vi "reward_behavior_phase1.vi"() -> ()   [LabVIEW 2019]
doc: "The myRIO Project template acquires acceleration data from the onboard accelerometer and displays the changes of acceleration values in a waveform chart."
uses:
  <vilib>/Analysis/Matrix/Datatypes/RealMatrix.ctl
  <vilib>/myRIO/Common/Instrument Driver Framework/myRIO v1.0/Encoder/typedefs/Encoder Signal Mode.ctl
  <vilib>/myRIO/Instrument Drivers/Onboard IO/Encoder/typedefs/Encoder Reference.ctl
  <vilib>/myRIO/Common/Instrument Driver Framework/Utilities/typedefs/myRIO Generic Hardware Reference.ctl
  <vilib>/myRIO/Common/Instrument Driver Framework/Utilities/typedefs/Hardware Version Enum.ctl
  <vilib>/myRIO/Common/Instrument Driver Framework/Utilities/typedefs/myRIO v1.0 Reference.ctl
  <vilib>/myRIO/Common/Instrument Driver Framework/Utilities/typedefs/Generic FPGA Reference.ctl
  <vilib>/myRIO/Common/Instrument Driver Framework/myRIO v1.0/Encoder/typedefs/Encoder Channels Enum.ctl
  <vilib>/myRIO/Common/Instrument Driver Framework/myRIO v1.0/Encoder/typedefs/Encoder Configuration v1.0.ctl
  <vilib>/userdefined/High Color/nirio_resource_hc.ctl
  <vilib>/myRIO/Instrument Drivers/Onboard IO/DIO/typedefs/DIO Reference.ctl
  <vilib>/myRIO/Common/Instrument Driver Framework/myRIO v1.0/DIO/typedefs/DIO Channels List.ctl
  <vilib>/myRIO/Common/Instrument Driver Framework/myRIO v1.0/DIO/typedefs/DIO Channels Enum.ctl
  <vilib>/myRIO/Common/Instrument Driver Framework/Utilities/vis/Is FPGA Ref Available.vi
  <vilib>/myRIO/Common/Instrument Driver Framework/myRIO v1.0/Encoder/vis/myRIO v1.1 Open Encoder.vi
  <vilib>/myRIO/Instrument Drivers/Onboard IO/Encoder/vis/Read.vi
  <vilib>/myRIO/Common/Instrument Driver Framework/myRIO v1.0/DIO/vis/myRIO v1.1 Open DIO.vi
  <vilib>/myRIO/Instrument Drivers/Onboard IO/DIO/vis/Write.vi
  <vilib>/myRIO/Instrument Drivers/Onboard IO/DIO/vis/Read.vi
  <vilib>/myRIO/Common/Instrument Driver Framework/Utilities/vis/Validate Channels.vi
  <vilib>/myRIO/Common/Instrument Driver Framework/myRIO v1.0/Encoder/vis/myRIO v1.0 Reserve Encoder.vi
  <vilib>/myRIO/Common/Instrument Driver Framework/myRIO v1.0/DIO/vis/myRIO v1.0 Reserve DIO.vi
  <vilib>/myRIO/Common/Instrument Driver Framework/myRIO v1.0/Encoder/vis/myRIO v1.0 Build MUX Configuration Encoder.vi
  <vilib>/myRIO/Common/Instrument Driver Framework/myRIO v1.0/Resource Manager/vis/myRIO v1.0 Reserve Channel List.vi
  <vilib>/myRIO/Common/Instrument Driver Framework/myRIO v1.0/DIO/vis/myRIO v1.0 Build MUX Configuration DIO.vi
  <vilib>/myRIO/Common/Instrument Driver Framework/myRIO v1.0/Resource Manager/vis/myRIO v1.0 Create Configuration List.vi
  <vilib>/myRIO/Common/Instrument Driver Framework/myRIO v1.0/Resource Manager/vis/myRIO v1.0 Reserve Channel.vi
  <vilib>/myRIO/Common/Instrument Driver Framework/myRIO v1.0/Resource Manager/vis/myRIO v1.0 Unreserve Channel.vi
  <vilib>/myRIO/Common/Instrument Driver Framework/myRIO v1.0/Resource Manager/vis/myRIO v1.0 Build Mutex Name.vi
  <vilib>/Utility/VariantDataType/GetNumericInfo.vi
  <vilib>/Utility/error.llb/Error Cluster From Error Code.vi
  <vilib>/myRIO/Common/Instrument Driver Framework/myRIO v1.0/myRIO v1.1 Open.vi
  <vilib>/myRIO/Common/Instrument Driver Framework/Utilities/vis/IO Manager.vi
  <vilib>/myRIO/Common/Instrument Driver Framework/Utilities/vis/Configuration Manager.vi
  <vilib>/myRIO/Common/Instrument Driver Framework/myRIO v1.0/Resource Manager/vis/myRIO v1.0 Configure IO.vi
  <vilib>/myRIO/Common/Instrument Driver Framework/myRIO v1.0/myRIO v1.0 Close.vi
  <vilib>/myRIO/Common/Instrument Driver Framework/myRIO v1.0/Encoder/vis/myRIO v1.0 Configure Encoder.vi
  <vilib>/myRIO/Common/Instrument Driver Framework/myRIO v1.0/Encoder/vis/myRIO v1.0 Read Encoder.vi
  <vilib>/myRIO/Common/Instrument Driver Framework/myRIO v1.0/DIO/vis/myRIO v1.0 Read DIO.vi
  <vilib>/myRIO/Common/Instrument Driver Framework/myRIO v1.0/DIO/vis/myRIO v1.0 Write DIO.vi
  <vilib>/myRIO/Express VI/Onboard IO/Encoder/Encoder Express VI.xnode
  <vilib>/myRIO/Instrument Drivers/Onboard IO/Encoder/vis/myRIO Encoder Open.xnode
  <vilib>/myRIO/Express VI/Onboard IO/DI/DI Express VI.xnode
  <vilib>/myRIO/Instrument Drivers/Onboard IO/DIO/vis/myRIO DIO Open.xnode
  <vilib>/myRIO/Express VI/Onboard IO/DO/DO Express VI.xnode
  <vilib>/myRIO/Instrument Drivers/Onboard IO/Encoder/Encoder.lvlib
  <vilib>/myRIO/Instrument Drivers/Onboard IO/DIO/DIO.lvlib
  <vilib>/Analysis/Matrix/NI_Matrix.lvlib
panel:
  out "Rewarded trials":dbl[](array[numeric])
  out "Rewards":u16
  out "Active Trial":bool
  out "Array temp2":T1
  out "Stimuli Loaded":bool
  out "Stim_ID":dbl[](array[numeric])
  out "Reward_mat":dbl[](array[numeric])
  out "Reward":bool=TRUE
  out "Frame clock":i32
  out "Licks":u32
  out "Lick":bool
  out "Time":dbl
  out "Stop":bool
  in  "Frames to collect":u32
  out "Overflow?":bool
  out "Counter Value":i32
  out "Velocity":dbl
  out "Velocity Plot":dbl[](graph)
  out "Velocity array":dbl[](array[numeric])
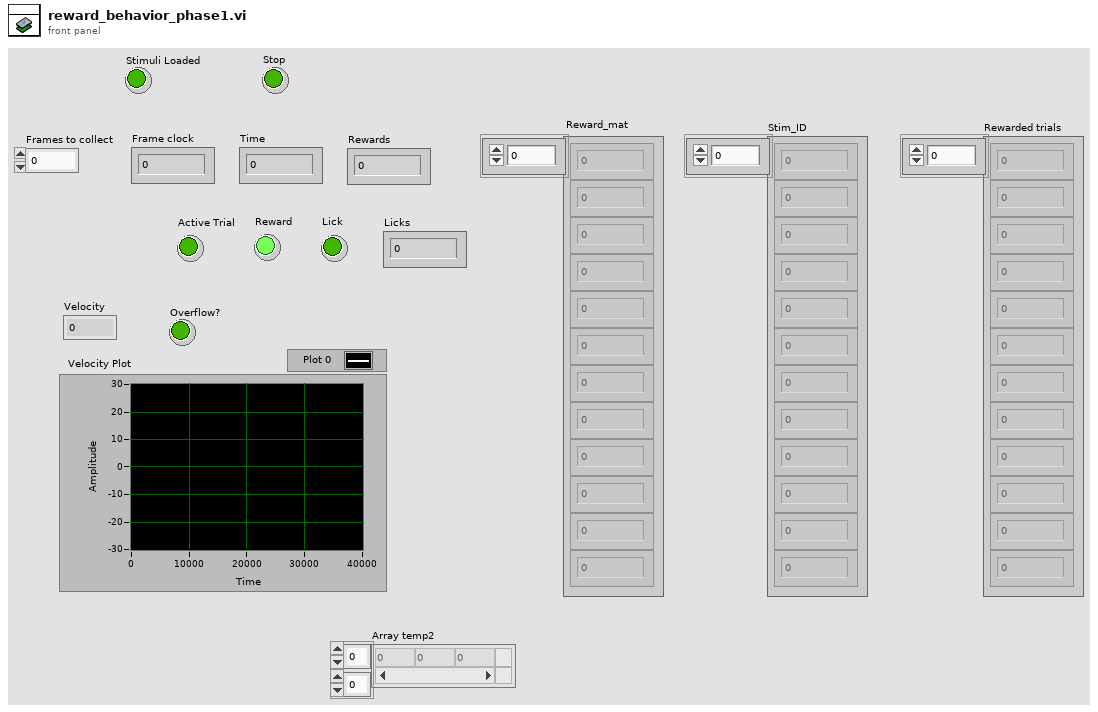
[diagram p1: front panel]
types:
  T1 = typedef "NI_Matrix.lvlib/RealMatrix.ctl" = dbl[][]
  T2 = typedef "Encoder.lvlib/Encoder Reference.ctl" = cluster{"myRIO Reference":T3, "Encoder Channels Enum":T7}
  T3 = typedef "myRIO Generic Hardware Reference.ctl" = cluster{"myRIO Model":T4, "myRIO Hardware Reference":T5}
  T4 = typedef "Hardware Version Enum.ctl" = enum16{"Unknown", "myRIO-1900", "myRIO-1950", "roboRIO", "NI ELVIS RIO CM", "ELVIS III"}
  T5 = typedef "myRIO v1.0 Reference.ctl" = cluster{"Generic FPGA Reference":T6, "Allow multiple opens":bool}
  T6 = typedef "Generic FPGA Reference.ctl" = refnum<k20>
  T7 = typedef "Encoder Channels Enum.ctl" = enum16{"Not Connected", "C/ENC0", "C/ENC1", "A/ENC", "A/ENC0", "A/ENC1", "A/ENC2", "A/ENC3", "A/ENC4", "A/ENC5", "A/ENC6", "A/ENC7", "A/ENC8", "A/ENC9", "B/ENC", "B/ENC0", "B/ENC1", "B/ENC2", "B/ENC3", "B/ENC4", "B/ENC5", "B/ENC6", "B/ENC7", "B/ENC8", "B/ENC9", "DIO/ENC0", "DIO/ENC1", "DIO/ENC2", "DIO/ENC3", "DIO/ENC4"}
  T8 = typedef "Encoder Signal Mode.ctl" = enum16{"Quadrature phase signal", "Step and direction signal"}
  T9 = typedef "nirio_resource_hc.ctl" = tag
  T10 = typedef "DIO.lvlib/DIO Reference.ctl" = cluster{"myRIO Reference":T3, "DIO Channels List":T11}
  T11 = typedef "DIO Channels List.ctl" = T12[]
  T12 = typedef "DIO Channels Enum.ctl" = enum16{"Not Connected", "C/DIO0", "C/DIO1", "C/DIO2", "C/DIO3", "C/DIO4", "C/DIO5", "C/DIO6", "C/DIO7", "A/DIO0", "A/DIO1", "A/DIO2", "A/DIO3", "A/DIO4", "A/DIO5", "A/DIO6", "A/DIO7", "A/DIO8", "A/DIO9", "A/DIO10", "A/DIO11", "A/DIO12", "A/DIO13", "A/DIO14", "A/DIO15", "A/DIO16", "A/DIO17", "A/DIO18", "A/DIO19", "B/DIO0", "B/DIO1", "B/DIO2", "B/DIO3", "B/DIO4", "B/DIO5", "B/DIO6", "B/DIO7", "B/DIO8", "B/DIO9", "B/DIO10", "B/DIO11", "B/DIO12", "B/DIO13", "B/DIO14", "B/DIO15", "B/DIO16", "B/DIO17", "B/DIO18", "B/DIO19", "LED0", "LED1", "LED2", "LED3", "Button0", "DIO/DIO0", "DIO/DIO1", "DIO/DIO2", "DIO/DIO3", "DIO/DIO4", "DIO/DIO5", "DIO/DIO6", "DIO/DIO7", "DIO/DIO8", "DIO/DIO9", "SPI/CS0", "SPI/CS1", "SPI/CS2", "SPI/CS3", "LED RADIO (Green)", "LED RADIO (Red)", "LED COMM (Green)", "LED COMM (Red)", "LED MODE (Green)", "LED MODE (Red)"}
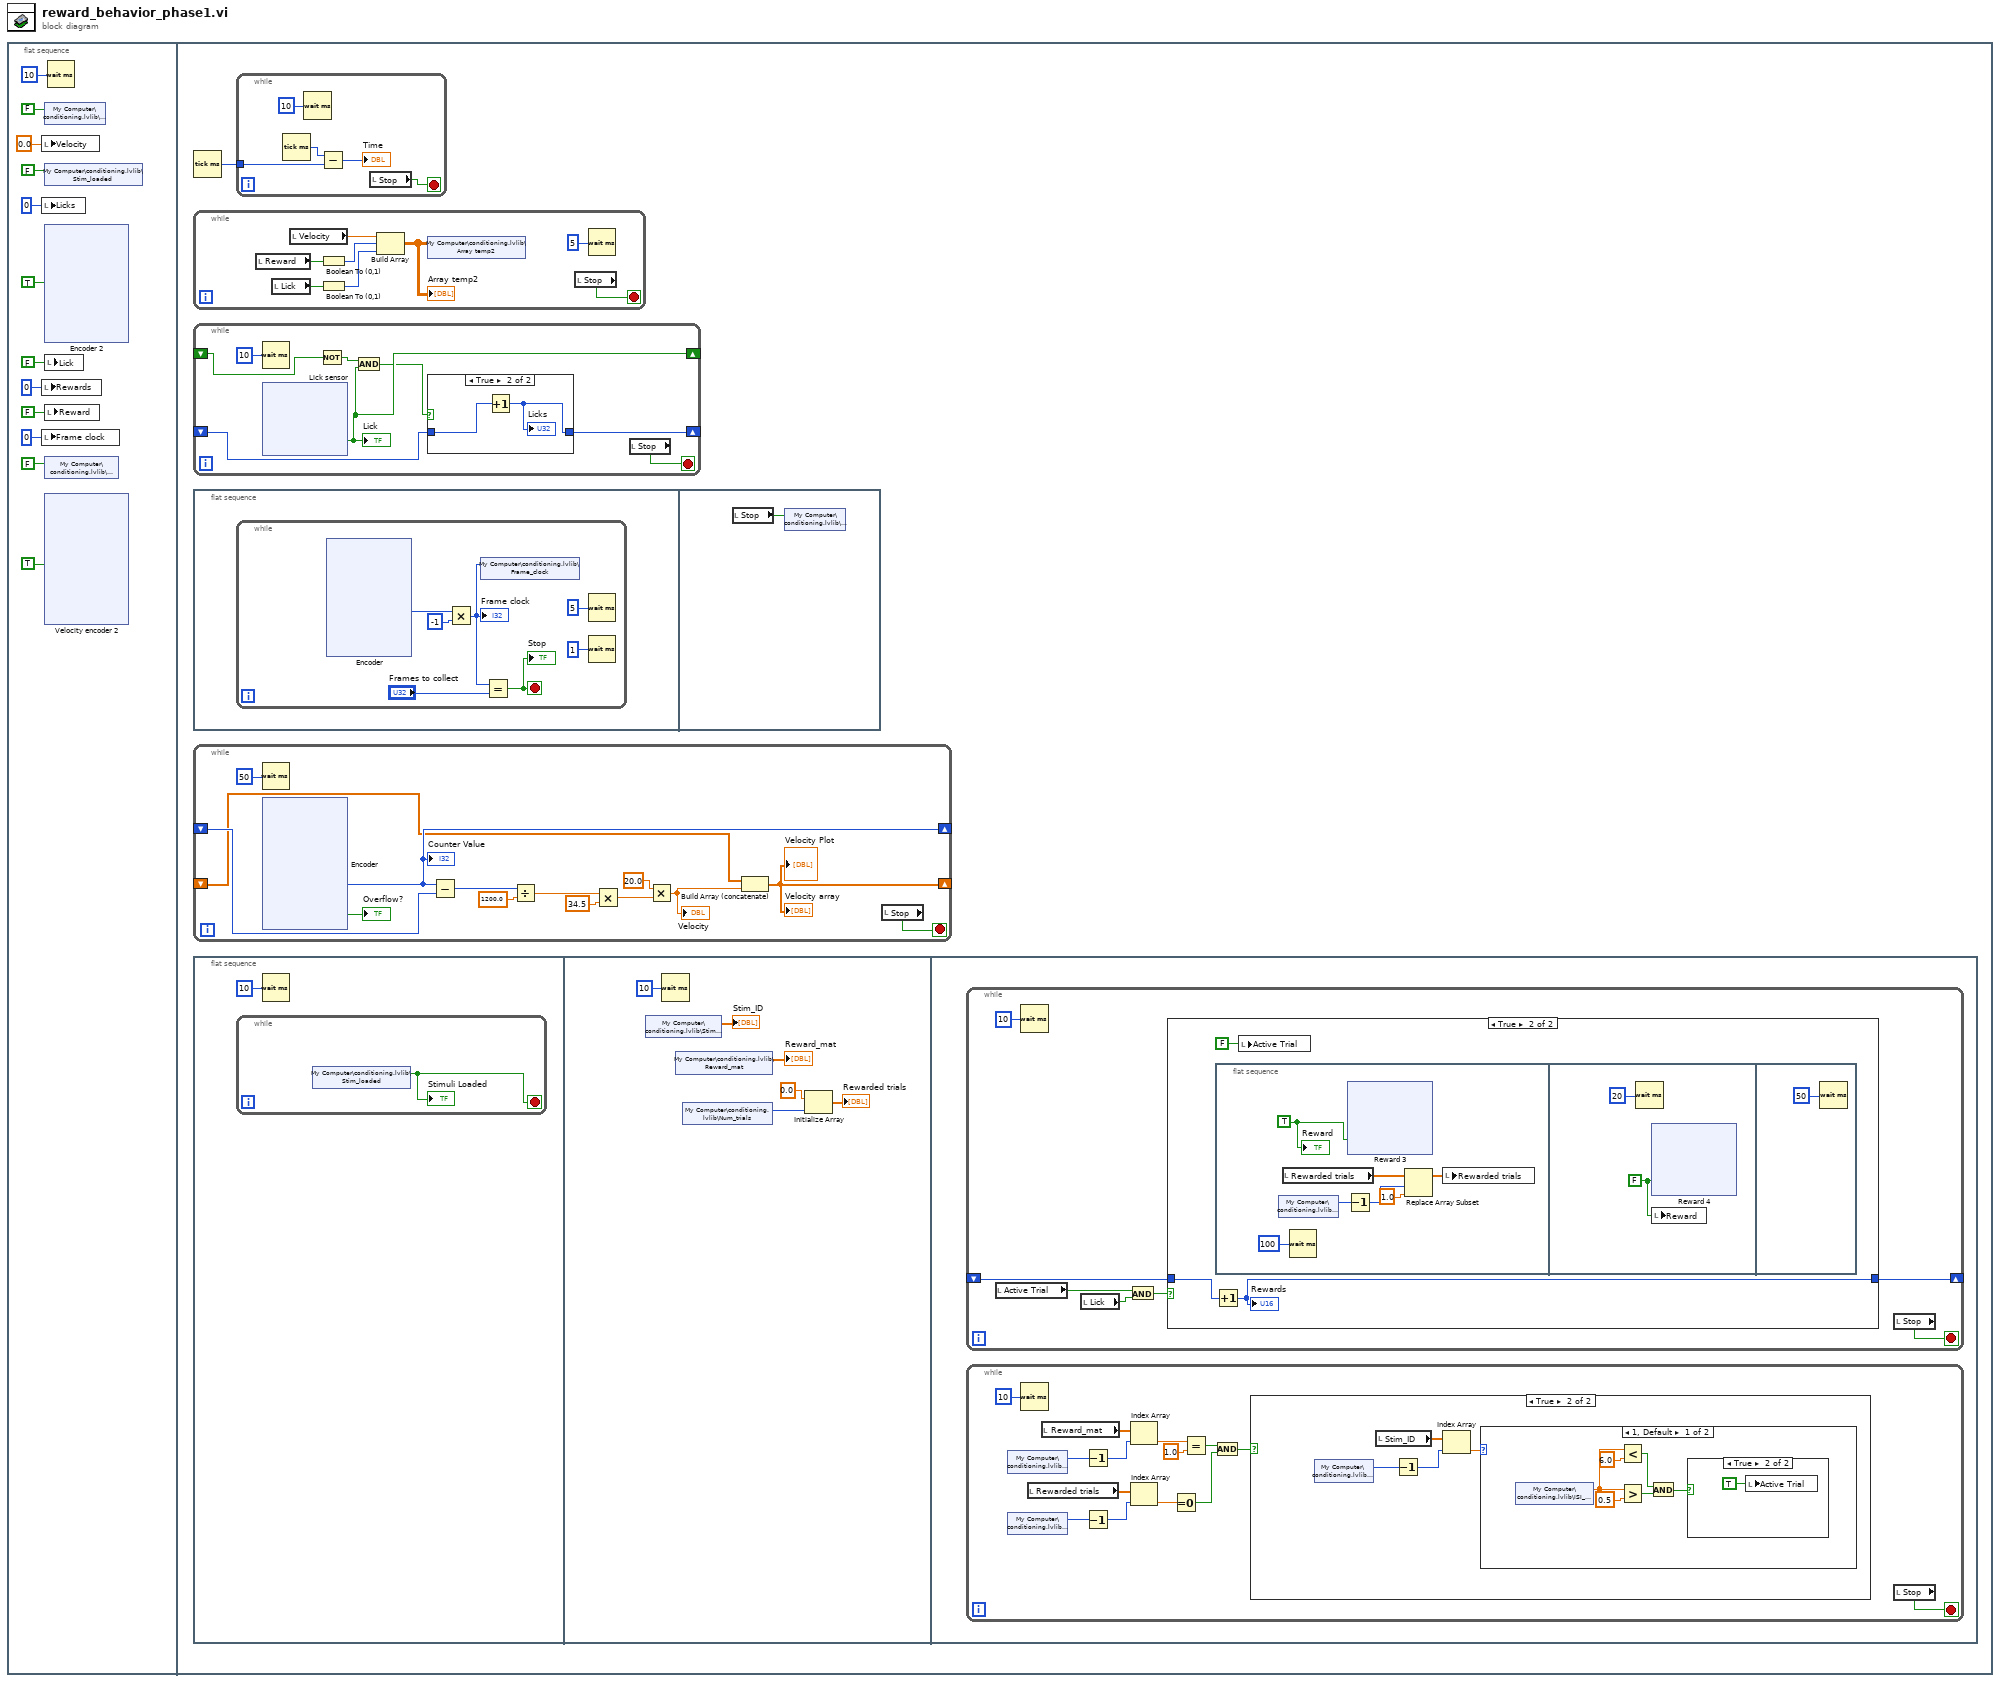
[diagram p0: block diagram]
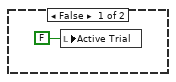
[diagram p2: hidden frame]
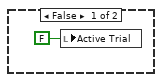
[diagram p3: hidden frame]
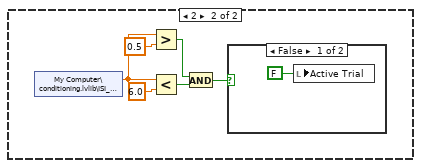
[diagram p4: hidden frame]
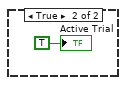
[diagram p5: hidden frame]
diagram:
  n1 = flat-sequence {
    frame #0 {
      n2 = local write "Velocity"(0.0 ("Velocity")) -> ()
      n3 = local write "Licks"(u32 0 ("Licks")) -> ()
      n4 = local write "Rewards"(u16 0 ("Rewards")) -> ()
      n5 = local write "Frame clock"(u32 0 ("Frames")) -> ()
      n6 = shared-variable "My Computer\\conditioning.lvlib\\Stop"(FALSE ("Stop")) -> ()  [unwired: 1 in, 1 out]
      n7 = shared-variable "My Computer\\conditioning.lvlib\\Stim_loaded"(FALSE ("Stim_loaded")) -> ()  [unwired: 1 in, 1 out]
      n8 = xnode "Encoder 2"("Reset Counter"=TRUE) -> ()  [unwired: 1 in, 4 out]
      n9 = local write "Lick"(FALSE ("Lick")) -> ()
      n10 = local write "Reward"(FALSE ("Give reward")) -> ()
      n11 = shared-variable "My Computer\\conditioning.lvlib\\Display"(FALSE ("Display")) -> ()  [unwired: 1 in, 1 out]
      n12 = xnode "Velocity encoder 2"("Reset Counter"=TRUE) -> ()  [unwired: 1 in, 4 out]
      n13 = Wait (ms)(milliseconds to wait=u32 10) -> ()  [unwired: 1 out]
    }
    frame #1 {
      n14 = Tick Count (ms)() -> (millisecond timer value=w105:u32)
      n15 = while {
        stop <- w107 stop-if-true
        n16 = local read "Reward"() -> (w112:bool)
        n17 = local read "Lick"() -> (w113:bool)
        n18 = local read "Velocity"() -> (w111:dbl)
        n19 = Boolean To (0,1)(Boolean=w112) -> (0, 1=w110:i16)
        n20 = Boolean To (0,1)(Boolean=w113) -> (0, 1=w109:i16)
        n21 = Build Array(w111, w110, w109) -> (w106:T1)
        "Array temp2" <- w106
        n22 = shared-variable "My Computer\\conditioning.lvlib\\Array temp2"(w106) -> ()  [unwired: 1 in, 1 out]
        n23 = local read "Stop"() -> (w107:bool)
        n24 = Wait (ms)(milliseconds to wait=u32 5) -> ()  [unwired: 1 out]
      }
      n25 = while {
        shift-right: [w308] -> _
        shift-left: _ -> [w307]
        shift-right: [w303] -> _
        shift-left: _ -> [w305]
        stop <- w306 stop-if-true
        n26 = Wait (ms)(milliseconds to wait=u32 10) -> ()  [unwired: 1 out]
        n27 = xnode "Lick sensor"() -> ("C/DIO1 (DIO1)"=w303:bool)  [unwired: 1 in, 1 out]
        "Lick" <- w303
        n28 = Not(x=w305) -> (.not. x?=w304:bool)
        n29 = And(x=w304, y=w303) -> (x .and. y?=w302:bool)
        n30 = case shown="True" w302 {
          tunnel: [w310 w312] -> w308
          tunnel: w307 -> [w310 w311]
          frame False {
          }
          frame True {
            n31 = Increment(x=w311) -> (x+1=w312:u32)
            "Licks" <- w312
          }
        }
        n32 = local read "Stop"() -> (w306:bool)
      }
      n33 = flat-sequence {
        frame #0 {
          n34 = while {
            stop <- w249 stop-if-true
            n35 = xnode "Encoder"() -> ("Counter Value"=w253:i32)  [unwired: 2 in, 3 out]
            n36 = Multiply(x=w253, y=-1) -> (x*y=w248:i32)
            "Frame clock" <- w248
            n37 = shared-variable "My Computer\\conditioning.lvlib\\Frame_clock"(w248) -> ()  [unwired: 1 in, 1 out]
            n38 = Equal?(x=w248, y="Frames to collect") -> (x = y?=w249:bool)
            "Stop" <- w249
            n39 = Wait (ms)(milliseconds to wait=u32 5) -> ()  [unwired: 1 out]
            n40 = Wait (ms)(milliseconds to wait=u32 1) -> ()  [unwired: 1 out]
          }
        }
        frame #1 {
          n41 = local read "Stop"() -> (w301:bool)
          n42 = shared-variable "My Computer\\conditioning.lvlib\\Stop"(w301) -> ()  [unwired: 1 in, 1 out]
        }
      }
      n43 = while {
        shift-right: [w358] -> _
        shift-left: _ -> [w359]
        shift-right: [w350] -> _
        shift-left: _ -> [w349]
        stop <- w348 stop-if-true
        n44 = Wait (ms)(milliseconds to wait=u32 50) -> ()  [unwired: 1 out]
        n45 = xnode "Encoder"() -> ("Counter Value"=w358:i32, "Overflow?"=→"Overflow?":bool)  [unwired: 2 in, 2 out]
        "Counter Value" <- w358
        n46 = Subtract(x=w358, y=w359) -> (x-y=w351:i32)
        n47 = Divide(x=w351, y=1200.0 ("600")) -> (x/y=w356:dbl)
        n48 = Multiply(x=w356, y=34.5) -> (x*y=w354:dbl)
        n49 = Multiply(x=20.0, y=w354) -> (x*y=w352:dbl)
        "Velocity" <- w352
        n50 = Build Array (concatenate)(w349, w352) -> (w350:dbl[])
        "Velocity Plot" <- w350
        "Velocity array" <- w350
        n51 = local read "Stop"() -> (w348:bool)
      }
      n52 = flat-sequence {
        frame #0 {
          n53 = while {
            stop <- w115 stop-if-true
            n54 = shared-variable "My Computer\\conditioning.lvlib\\Stim_loaded"() -> (w115:bool)  [unwired: 1 in, 1 out]
            "Stimuli Loaded" <- w115
          }
          n55 = Wait (ms)(milliseconds to wait=u32 10) -> ()  [unwired: 1 out]
        }
        frame #1 {
          n56 = shared-variable "My Computer\\conditioning.lvlib\\Stim_ID"() -> (→"Stim_ID":dbl[])  [unwired: 1 in, 1 out]
          n57 = Wait (ms)(milliseconds to wait=u32 10) -> ()  [unwired: 1 out]
          n58 = shared-variable "My Computer\\conditioning.lvlib\\Reward_mat"() -> (→"Reward_mat":dbl[])  [unwired: 1 in, 1 out]
          n59 = shared-variable "My Computer\\conditioning.lvlib\\Num_trials"() -> (w118:u32)  [unwired: 1 in, 1 out]
          n60 = Initialize Array(0.0 ("element"), w118) -> (→"Rewarded trials":dbl[])
        }
        frame #2 {
          n61 = while {
            shift-right: [w160] -> _
            shift-left: _ -> [w159]
            stop <- w163 stop-if-true
            n62 = local read "Active Trial"() -> (w157:bool)
            n63 = Wait (ms)(milliseconds to wait=u32 10) -> ()  [unwired: 1 out]
            n64 = local read "Lick"() -> (w158:bool)
            n65 = And(x=w157, y=w158) -> (x .and. y?=w161:bool)
            n66 = case shown="True" w161 {
              tunnel: [w164 w167] -> w160
              tunnel: w159 -> [w164 w166]
              frame False {
              }
              frame True {
                n67 = Increment(x=w166) -> (x+1=w167:u16)
                "Rewards" <- w167
                n68 = flat-sequence {
                  frame #0 {
                    w173 = TRUE ("C/DIO0 (DIO0)")
                    n69 = shared-variable "My Computer\\conditioning.lvlib\\Trial"() -> (w172:u32)  [unwired: 1 in, 1 out]
                    n70 = local read "Rewarded trials"() -> (w170:dbl[])
                    n71 = Wait (ms)(milliseconds to wait=u32 100) -> ()  [unwired: 1 out]
                    n72 = Decrement(x=w172) -> (x-1=w171:u32)
                    n73 = xnode "Reward 3"("C/DIO0 (DIO0)"=w173) -> ()  [unwired: 1 in, 1 out]
                    n74 = Replace Array Subset(array=w170, new element=1.0 ("new element/subarray"), index=w171) -> (w168:dbl[])
                    n75 = local write "Rewarded trials"(w168) -> ()
                    "Reward" <- w173
                  }
                  frame #1 {
                    w211 = FALSE ("C/DIO0 (DIO0)")
                    n76 = Wait (ms)(milliseconds to wait=u32 20) -> ()  [unwired: 1 out]
                    n77 = xnode "Reward 4"("C/DIO0 (DIO0)"=w211) -> ()  [unwired: 1 in, 1 out]
                    n78 = local write "Reward"(w211) -> ()
                  }
                  frame #2 {
                    n79 = Wait (ms)(milliseconds to wait=u32 50) -> ()  [unwired: 1 out]
                  }
                }
                n80 = local write "Active Trial"(FALSE ("Active Trial")) -> ()
              }
            }
            n81 = local read "Stop"() -> (w163:bool)
          }
          n82 = while {
            stop <- w135 stop-if-true
            n83 = shared-variable "My Computer\\conditioning.lvlib\\Trial"() -> (w131:u32)  [unwired: 1 in, 1 out]
            n84 = shared-variable "My Computer\\conditioning.lvlib\\Trial"() -> (w127:u32)  [unwired: 1 in, 1 out]
            n85 = Wait (ms)(milliseconds to wait=u32 10) -> ()  [unwired: 1 out]
            n86 = local read "Rewarded trials"() -> (w128:dbl[])
            n87 = local read "Reward_mat"() -> (w130:dbl[])
            n88 = Decrement(x=w131) -> (x-1=w132:u32)
            n89 = Decrement(x=w127) -> (x-1=w126:u32)
            n90 = Index Array(array=w130, index=w132) -> (element=w133:dbl)
            n91 = Index Array(array=w128, index=w126) -> (element=w125:dbl)
            n92 = Equal To 0?(x=w125) -> (x = 0?=w124:bool)
            n93 = Equal?(x=w133, y=1.0) -> (x = y?=w123:bool)
            n94 = And(x=w123, y=w124) -> (x .and. y?=w122:bool)
            n95 = case shown="True" w122 {
              frame False {
                n96 = local write "Active Trial"(FALSE ("Active_trial")) -> ()
              }
              frame True {
                n97 = shared-variable "My Computer\\conditioning.lvlib\\Trial"() -> (w138:u32)  [unwired: 1 in, 1 out]
                n98 = local read "Stim_ID"() -> (w140:dbl[])
                n99 = Decrement(x=w138) -> (x-1=w139:u32)
                n100 = Index Array(array=w140, index=w139) -> (element=w137:dbl)
                n101 = case shown="1, Default" w137 {
                  frame 1, Default {
                    n102 = shared-variable "My Computer\\conditioning.lvlib\\ISI_Time"() -> (w145:dbl)  [unwired: 1 in, 1 out]
                    n103 = Less?(x=w145, y=6.0) -> (x < y?=w143:bool)
                    n104 = Greater?(x=w145, y=0.5) -> (0:w142:bool)
                    n105 = And(x=w143, y=w142) -> (x .and. y?=w141:bool)
                    n106 = case shown="True" w141 {
                      frame False {
                        n107 = local write "Active Trial"(FALSE ("Active Trial")) -> ()
                      }
                      frame True {
                        n108 = local write "Active Trial"(TRUE ("Active Trial")) -> ()
                      }
                    }
                  }
                  frame 2 {
                    n109 = shared-variable "My Computer\\conditioning.lvlib\\ISI_Time"() -> (w153:dbl)  [unwired: 1 in, 1 out]
                    n110 = Greater?(x=w153, y=0.5) -> (0:w151:bool)
                    n111 = Less?(x=w153, y=6.0) -> (x < y?=w150:bool)
                    n112 = And(x=w151, y=w150) -> (x .and. y?=w149:bool)
                    n113 = case shown="False" w149 {
                      frame False {
                        n114 = local write "Active Trial"(FALSE ("Active Trial")) -> ()
                      }
                      frame True {
                        "Active Trial" <- TRUE ("Active Trial")
                      }
                    }
                  }
                }
              }
            }
            n115 = local read "Stop"() -> (w135:bool)
          }
        }
      }
      n116 = while {
        tunnel: w105 -> [w411]
        stop <- w408 stop-if-true
        n117 = Tick Count (ms)() -> (millisecond timer value=w412:u32)
        n118 = Wait (ms)(milliseconds to wait=u32 10) -> ()  [unwired: 1 out]
        n119 = Subtract(x=w412, y=w411) -> (x-y=→"Time":u32)
        n120 = local read "Stop"() -> (w408:bool)
      }
    }
  }
